vi "Setup UI.vi"(8 "error in (no error)":errorcluster, 10 "Set UI to input? (F)":bool, 11 "Double Scanner in":refnum<class "Double Scanner.lvclass">) -> (0 "error out":errorcluster, 3 "Double Scanner out":refnum<class "Double Scanner.lvclass">)   [LabVIEW 2023, in "Double Scanner.lvclass"]
doc: "Scanner::Setup is a constructor that has no parameters and faces the user. The Factory calls this VI to let the user configure this Scanner. It is dynamically dispatched in order to let the user choose the type as well as the options of the scanner."
uses:
  Double Scanner.lvclass
  Double Scanner.lvclass/Double Scanner.ctl
  Scanner/Scanner.lvclass
panel:
  in  "Tab Control":enum32{"Scanner 1", "Scanner 2"}(tab)
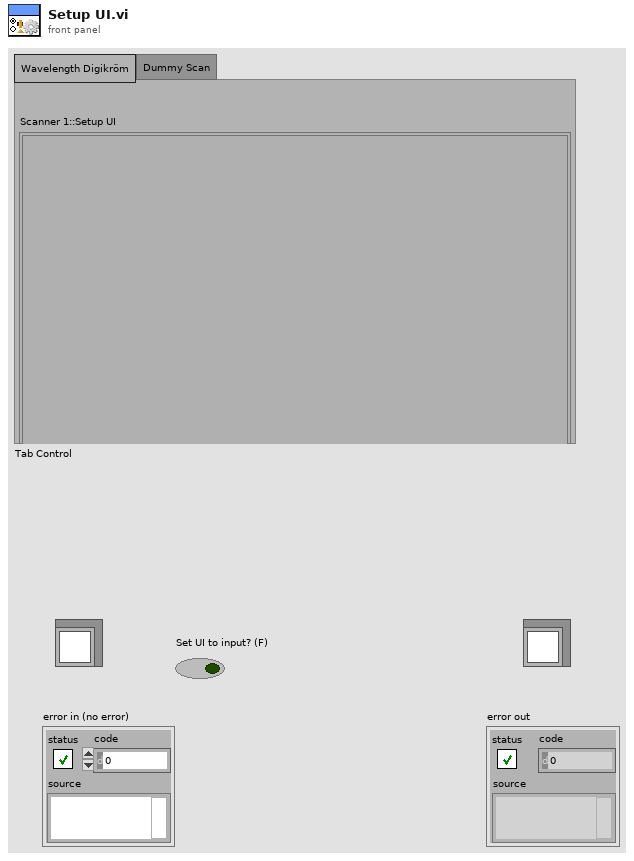
[diagram p1: front panel]
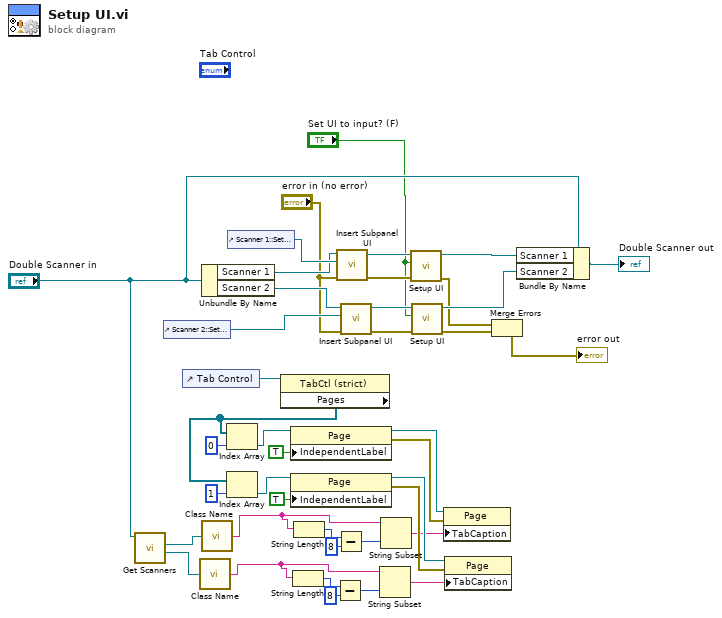
[diagram p0: block diagram]
diagram:
  n1 = call-dynamic "Get Scanners.vi"("Double Scanner in"="Double Scanner in") -> ("Scanner 2 out"=w35:refnum<class "Scanner.lvclass">, "Scanner 1 out"=w36:refnum<class "Scanner.lvclass">)  [unwired: 7 in, 2 out]
  n2 = control-ref of="Scanner 2::Setup UI"() -> (w38:refnum<vi>)
  n3 = control-ref of="Tab Control"() -> (w34:refnum<vi>)
  n4 = call "Class Name.vi"("LabVIEW Object"=w35) -> ("Class Name"=w15:string)
  n5 = Unbundle By Name("Double Scanner in") -> ("Scanner 1"=w40:refnum<class "Scanner.lvclass">, "Scanner 2"=w39:refnum<class "Scanner.lvclass">)
  n6 = call "Class Name.vi"("LabVIEW Object"=w36) -> ("Class Name"=w19:string)
  n7 = control-ref of="Scanner 1::Setup UI"() -> (w41:refnum<vi>)
  n8 = property class="TabCtl (strict)"(reference=w34) -> ("Pages"=w32:refnum<vi>[])  [unwired: 1 in, 2 out]
  n9 = Index Array(array=w32, index=0) -> (element=w29:refnum<vi>)
  n10 = Index Array(array=w32, index=1) -> (element=w30:refnum<vi>)
  n11 = property class="Page"(reference=w29, "IndependentLabel"=TRUE ("Independent Label")) -> (reference out=w25:refnum<vi>, error out=w24:errorcluster)  [unwired: 1 in]
  n12 = property class="Page"(reference=w30, "IndependentLabel"=TRUE ("Independent Label")) -> (reference out=w26:refnum<vi>, error out=w23:errorcluster)  [unwired: 1 in]
  n13 = String Length(string=w15) -> (length=w18:i32)
  n14 = String Length(string=w19) -> (length=w22:i32)
  n15 = Subtract(x=w18, y=8) -> (x-y=w16:i32)
  n16 = Subtract(x=w22, y=8) -> (x-y=w20:i32)
  n17 = call "Insert Subpanel UI.vi"("error in (no error)"="error in (no error)", "Subpanel in"=w41, "LabVIEW Object"=w40) -> ("error out"=w9:errorcluster, "LabVIEW Object out"=w11:refnum<class "Scanner.lvclass">)  [unwired: 7 out]
  n18 = call "Insert Subpanel UI.vi"("error in (no error)"="error in (no error)", "Subpanel in"=w38, "LabVIEW Object"=w39) -> ("error out"=w5:errorcluster, "LabVIEW Object out"=w6:refnum<class "Scanner.lvclass">)  [unwired: 7 out]
  n19 = String Subset(string=w15, length (rest)=w16) -> (substring=w13:string)  [unwired: 1 in]
  n20 = String Subset(string=w19, length (rest)=w20) -> (substring=w14:string)  [unwired: 1 in]
  n21 = call-dynamic "Setup UI.vi"("error in (no error)"=w9, "Set UI to input? (F)"="Set UI to input? (F)", "Scanner in"=w11) -> ("error out"=w3:errorcluster, "Scanner out"=w10:refnum<class "Scanner.lvclass">)  [unwired: 7 out]
  n22 = call-dynamic "Setup UI.vi"("error in (no error)"=w5, "Set UI to input? (F)"="Set UI to input? (F)", "Scanner in"=w6) -> ("error out"=w2:errorcluster, "Scanner out"=w4:refnum<class "Scanner.lvclass">)  [unwired: 7 out]
  n23 = property class="Page"(reference=w25, error in=w24, "TabCaption"=w14) -> ()  [unwired: 2 out]
  n24 = property class="Page"(reference=w26, error in=w23, "TabCaption"=w13) -> ()  [unwired: 2 out]
  n25 = Merge Errors(w3, w2) -> (→"error out":errorcluster)
  n26 = Bundle By Name(cluster="Double Scanner in", "Scanner 1"=w10, "Scanner 2"=w4) -> (→"Double Scanner out":refnum<class "Double Scanner.lvclass">)
